vi "PrepareInlineData.vi"(8 "error in (no error)":errorcluster, 10 "Inline Data":string, 11 "VI Refnum":refnum<vi>) -> (0 "error out":errorcluster, 1 "Control Data":map{string, variant}(c390), 2 "Data Name":string)   [LabVIEW 2019]
uses:
  65fd24c9-a785-4dc1-8b48-2da962c35a9e.vi
  d55797c9-58c8-4118-a156-a05c24b3ba98.vi
  <vilib>/JDP Science/JSONtext/Find Item.vi
  <vilib>/JDP Science/JSONtext/String Subset.vi
  <vilib>/JDP Science/JSONtext/Parsing/Parse Full Path or Item Name.vi
  <vilib>/JDP Science/JSONtext/Offset/Find Item Locations by Path.vi
  <vilib>/JDP Science/JSONtext/JSON text to Variant.vi
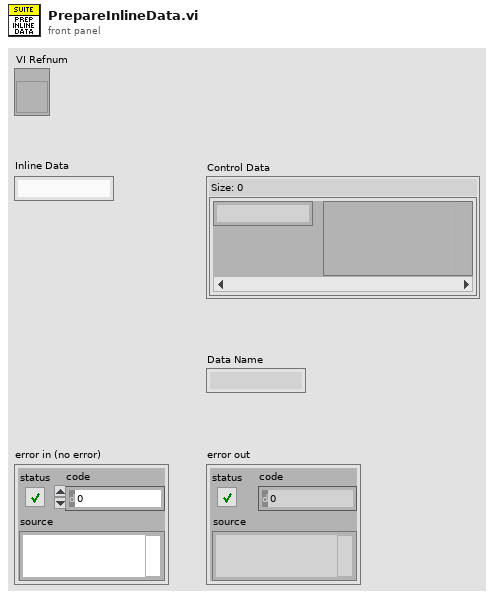
[diagram p1: front panel]
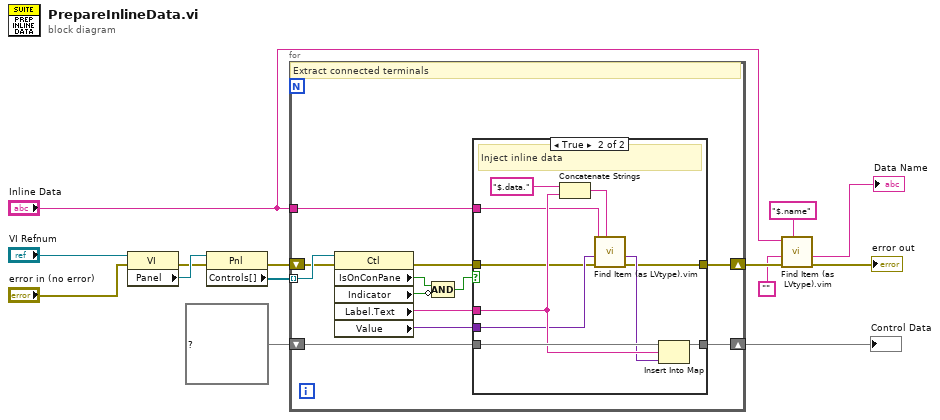
[diagram p0: block diagram]
diagram:
  n1 = property class="VI"(reference="VI Refnum", error in="error in (no error)") -> (error out=w13:errorcluster, "Panel"=w14:refnum<vi>)  [unwired: 1 out]
  n2 = property class="Pnl"(reference=w14, error in=w13) -> (error out=w11:errorcluster, "Controls[]"=w12:refnum<vi>[])  [unwired: 1 out]
  n3 = for {
    tunnel: w12 -> [w26] mode=indexing
    shift-right: [w18] -> w8
    shift-left: w11 -> [w25]
    shift-right: [w24] -> w2
    shift-left: map{string, variant} {} ("Controls") -> [w23]
    tunnel: "Inline Data" -> [w19]
    # "Extract connected terminals"
    n4 = property class="Ctl"(reference=w26, error in=w25) -> (error out=w20:errorcluster, "IsOnConPane"=w16:bool, "Indicator"=w17:bool, "Label.Text"=w22:string, "Value"=w21:variant)  [unwired: 1 out]
    n5 = Compound Arithmetic op=AND(w16, invert w17) -> (w15:bool)
    n6 = case shown="True" w15 {
      tunnel: [w28 w38] -> w24
      tunnel: w23 -> [w28 w37]
      tunnel: w22 -> [_ w34]
      tunnel: w21 -> [_ w33]
      tunnel: w20 -> [w27 w31]
      tunnel: [w27 w30] -> w18
      tunnel: w19 -> [_ w29]
      frame False {
      }
      frame True {
        # "Inject inline data"
        n7 = Concatenate Strings("$.data." ("string"), w34) -> (w36:string)
        n8 = call "Find Item (as LVtype).vim"("$Path or Item Name"=w36, "error in (no error)"=w31, "Data Type and Default Value"=w33, "JSON"=w29) -> ("error out"=w30:errorcluster, "Data"=w32:variant)  [unwired: 4 in, 2 out]
        n9 = Insert Into Map(map in=w37, key=w34, value=w32) -> (map out=w38:map{string, variant})  [unwired: 2 out]
      }
    }
  }
  "Control Data" <- w2
  n10 = call "Find Item (as LVtype).vim"("$Path or Item Name"="$.name", "error in (no error)"=w8, "Data Type and Default Value"="", "JSON"="Inline Data") -> ("error out"=→"error out":errorcluster, "Data"=→"Data Name":string)  [unwired: 4 in, 2 out]
